vi "GPS_DecimalDegreeToDegree.vi"(8 "error in (no error)":errorcluster caption="Fehler (Eingang, kein Fehler)", 9 "Lon(decimal degrees)":dbl=11.7335721 format="%.7f", 11 "Lat(decimal degrees)":dbl=48.1148849 format="%.7g") -> (0 "error out":errorcluster caption="Fehler (Ausgang)", 2 "GPS":string)   [LabVIEW 2017]
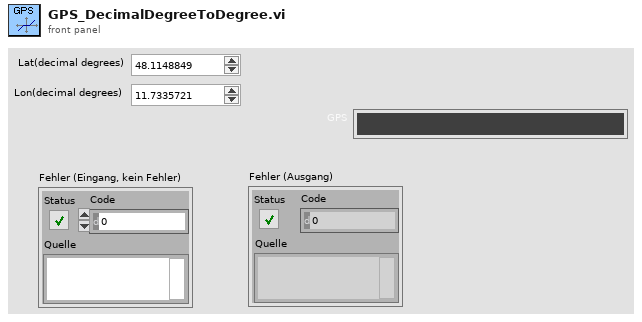
[diagram p1: front panel]
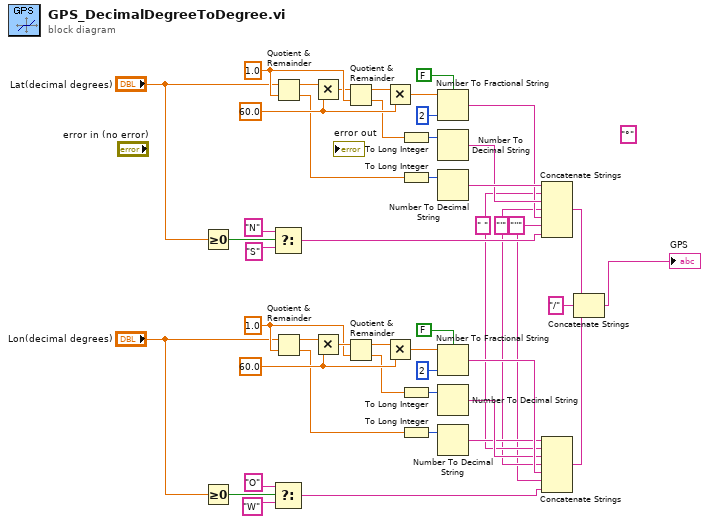
[diagram p0: block diagram]
diagram:
  (unwired) "°" ("String")
  w5 = "''" ("String")
  w6 = "'" ("String")
  w7 = " " ("String")
  w38 = 60.0 ("y")
  w39 = 1.0 ("y")
  w47 = 60.0 ("y")
  w46 = 1.0 ("y")
  n1 = Greater Or Equal To 0?(x="Lat(decimal degrees)") -> (x >= 0?=w26:bool)
  n2 = Greater Or Equal To 0?(x="Lon(decimal degrees)") -> (x >= 0?=w20:bool)
  n3 = Select(t="N" ("String"), s=w26, f="S" ("String")) -> (s? t:f=w23:string)
  n4 = Select(t="O" ("String"), s=w20, f="W" ("String")) -> (s? t:f=w8:string)
  n5 = Quotient & Remainder(x="Lat(decimal degrees)", y=w46) -> (x-y*floor(x/y)=w43:dbl, floor(x/y)=w30:dbl)
  n6 = Quotient & Remainder(x="Lon(decimal degrees)", y=w39) -> (x-y*floor(x/y)=w42:dbl, floor(x/y)=w11:dbl)
  n7 = Multiply(x=w43, y=w47) -> (x*y=w44:dbl)
  n8 = Multiply(x=w42, y=w38) -> (x*y=w41:dbl)
  n9 = Quotient & Remainder(x=w44, y=w46) -> (x-y*floor(x/y)=w45:dbl, floor(x/y)=w29:dbl)
  n10 = Quotient & Remainder(x=w41, y=w39) -> (x-y*floor(x/y)=w40:dbl, floor(x/y)=w10:dbl)
  n11 = Multiply(x=w45, y=w47) -> (x*y=w28:dbl)
  n12 = Multiply(x=w40, y=w38) -> (x*y=w12:dbl)
  n13 = To Long Integer(number=w29) -> (32bit integer=w37:i32)
  n14 = To Long Integer(number=w30) -> (32bit integer=w36:i32)
  n15 = To Long Integer(number=w10) -> (32bit integer=w13:i32)
  n16 = To Long Integer(number=w11) -> (32bit integer=w14:i32)
  n17 = Number To Fractional String(use system decimal point (T)=FALSE ("Systemdezimalzeichen verwenden (T)"), number=w28, precision (6)=i16 2 ("Genauigkeit (6)")) -> (F-format string=w32:string)  [unwired: 1 in]
  n18 = Number To Decimal String(number=w37) -> (decimal integer string=w34:string)  [unwired: 1 in]
  n19 = Number To Decimal String(number=w36) -> (decimal integer string=w35:string)  [unwired: 1 in]
  n20 = Number To Fractional String(use system decimal point (T)=FALSE ("Systemdezimalzeichen verwenden (T)"), number=w12, precision (6)=i16 2 ("Genauigkeit (6)")) -> (F-format string=w18:string)  [unwired: 1 in]
  n21 = Number To Decimal String(number=w13) -> (decimal integer string=w16:string)  [unwired: 1 in]
  n22 = Number To Decimal String(number=w14) -> (decimal integer string=w15:string)  [unwired: 1 in]
  n23 = Concatenate Strings(w35, w7, w34, w6, w32, w5, w23) -> (w4:string)
  n24 = Concatenate Strings(w15, w7, w16, w6, w18, w5, w8) -> (w3:string)
  n25 = Concatenate Strings(w4, "/" ("String"), w3) -> (→"GPS":string)
